vi "Set System Environment Variable.vi"(6 "Value":string, 7 "Environment Variable Name":string) -> ()   [LabVIEW 2017]
doc: "Sets a Windows environment variable for the current process and any child processes it starts."
uses:
  kernel32.dll
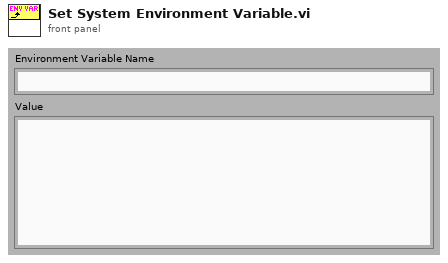
[diagram p1: front panel]
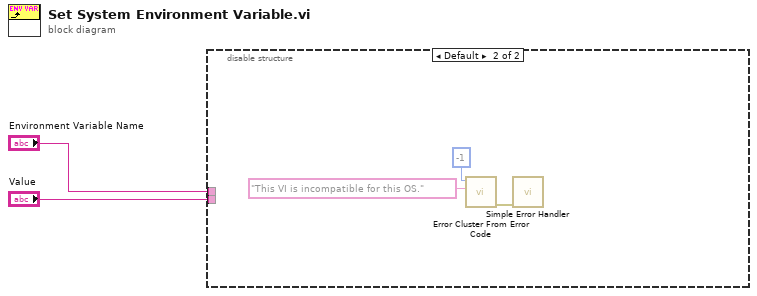
[diagram p0: block diagram]
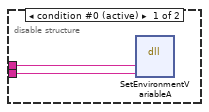
[diagram p2: hidden frame]
diagram:
  n1 = disable-structure shown="Default" {
    disable-tunnel: "Environment Variable Name" -> [w4 _]
    disable-tunnel: "Value" -> [w3 _]
    frame condition #0 (active) {
      n2 = dll-call lib="kernel32.dll" fn="SetEnvironmentVariableA"("EnvVarName"=w4, "Value"=w3) -> ()  [unwired: 6 in, 2 out]
    }
    frame condition #1 {
      n3 = call <vilib>:"Error Cluster From Error Code.vi"("error message (\"\")"="This VI is incompatible for this OS." ("error message (\"\")"), "error code (0)"=-1) -> ("error out"=w5:errorcluster)  [unwired: 7 in]
      n4 = call <vilib>:"Simple Error Handler.vi"("error in (no error)"=w5) -> ()  [unwired: 4 in, 5 out]
    }
  }
